vi "Spectrum.vi"() -> ()   [LabVIEW 2021]
uses:
  <userlib>/SciSDK/SciSDK_Labview.lvlib
panel:
  out "Valid Bins":u32
  out "Total Bins":u32
  out "Buffer Size":u32
  out "Integration time":u32
  out "Timecode":u32
  out "Magic":u32
  out "Histogram":i32[](graph)
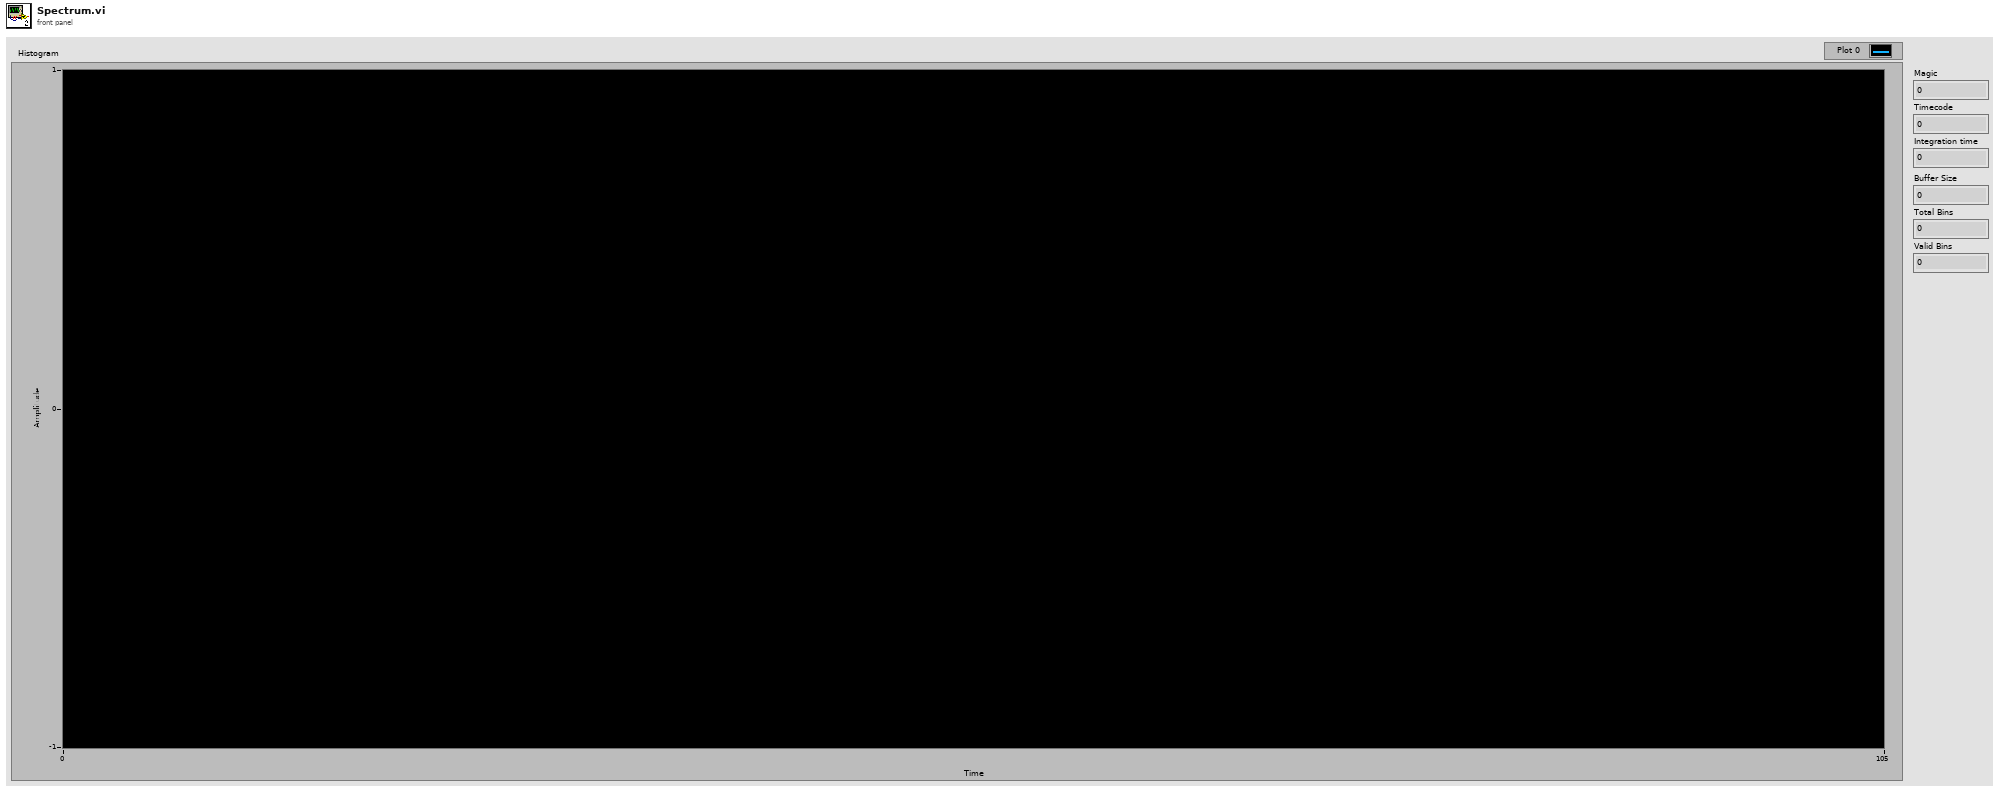
[diagram p1: front panel]
types:
  T1 = cluster{"Name":string, "Board Model":string, "Handle":u64}
  T2 = cluster{"Spectrum Path":string, "Spectrum Name":string}
  T3 = cluster{"magic":u32, "timecode":u32, "inttime":u32, "buffer_size":u32, "total_bins":u32, "valid_bins":u32, "data":i32[]}
  T4 = cluster{"Board Name":string, "Board Model":string, "Handle":u64}
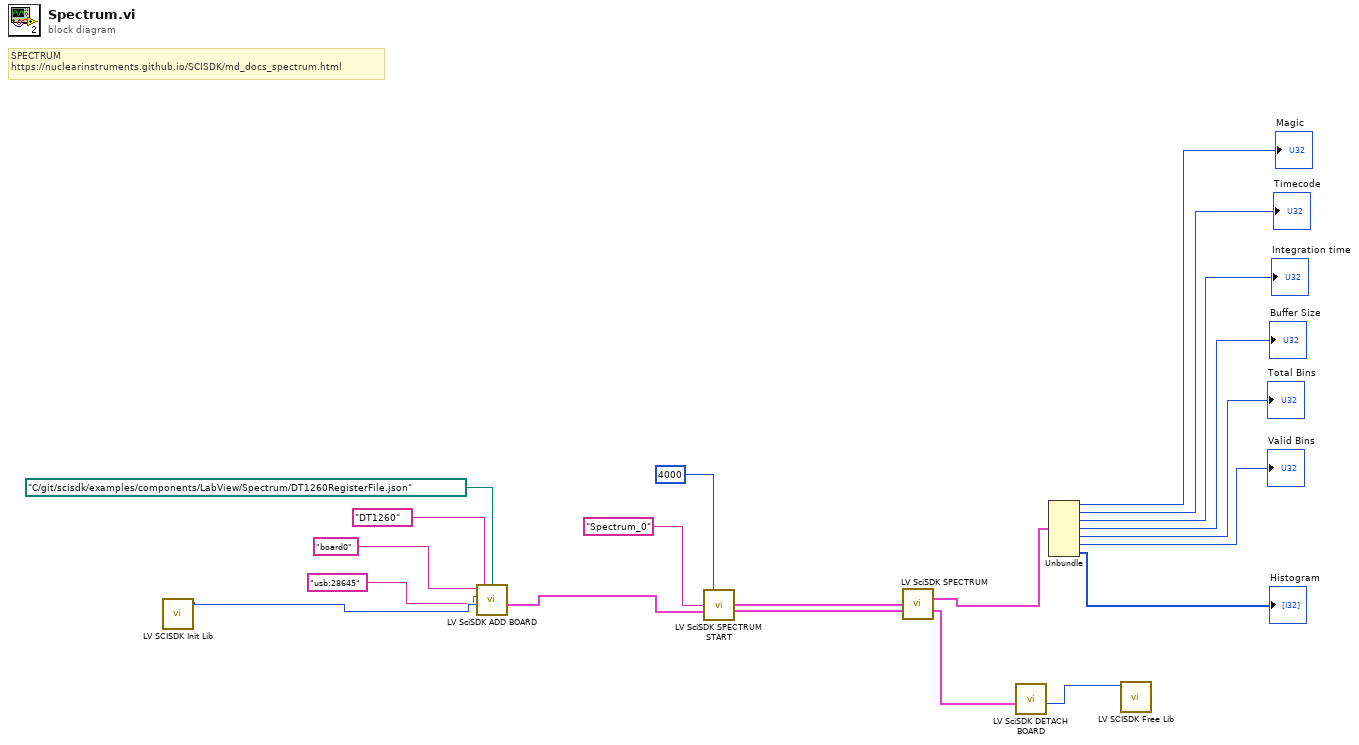
[diagram p0: block diagram]
diagram:
  # "SPECTRUM\nhttps://nuclearinstruments.github.io/SCISDK/md_docs_spectrum.html"
  n1 = call <userlib>:"LV SCISDK Init Lib.vi"() -> ("function return"=w13:u64)  [unwired: 11 in]
  n2 = call <userlib>:"LV SciSDK ADD BOARD.vi"("JsonFile"=path "C:/git/scisdk/examples/components/LabView/Spectrum/DT1260RegisterFile.json", "Board Model"="DT1260", "SciSDK Handle"=w13, "DevicePath"="usb:28645", "Name"="board0") -> ("Board Handle Out"=w7:T1)  [unwired: 4 in, 2 out]
  n3 = call <userlib>:"LV SciSDK SPECTRUM START.vi"("max"=u32 4000, "Spectrum name"="Spectrum_0", "Board Handle In"=w7) -> ("Handle Out"=w5:T2, "Board Handle Out"=w4:T1)  [unwired: 10 in, 1 out]
  n4 = call <userlib>:"LV SciSDK SPECTRUM.vi"("Spectrum Handle In"=w5, "Board Handle In"=w4) -> ("Spectrum Buffer Out"=w6:T3, "Board Handle Out"=w1:T4)  [unwired: 9 in, 3 out]
  n5 = call <userlib>:"LV SciSDK DETACH BOARD.vi"("Board Handle In"=w1) -> ("SciSDK Handle"=w2:u64)  [unwired: 9 in, 1 out]
  n6 = Unbundle(w6) -> ("magic"=→"Magic":u32, "timecode"=→"Timecode":u32, "inttime"=→"Integration time":u32, "buffer_size"=→"Buffer Size":u32, "total_bins"=→"Total Bins":u32, "valid_bins"=→"Valid Bins":u32, "data"=→"Histogram":i32[])
  n7 = call <userlib>:"LV SCISDK Free Lib.vi"("handle"=w2) -> ()  [unwired: 9 in, 2 out]
